vi "Read WebSocket.vi"(8 "error in (no error)":errorcluster, 11 "Connection Handler in":refnum<class "Connection Handler.lvclass">) -> (0 "error out":errorcluster, 2 "Socket":refnum<class "Socket.lvclass">, 3 "Connection Handler out":refnum<class "Connection Handler.lvclass">)   [LabVIEW 2017, in "Connection Handler.lvlib" / "Connection Handler.lvclass"]
uses:
  Connection Handler.lvclass
  <vilib>/MediaMongrels Ltd/WebSockets/Sockets/Socket/Socket.lvclass
  Connection Handler.lvclass/Connection Handler.ctl
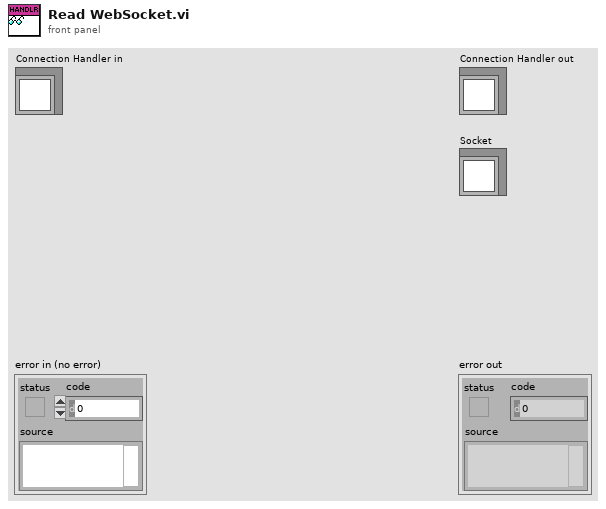
[diagram p1: front panel]
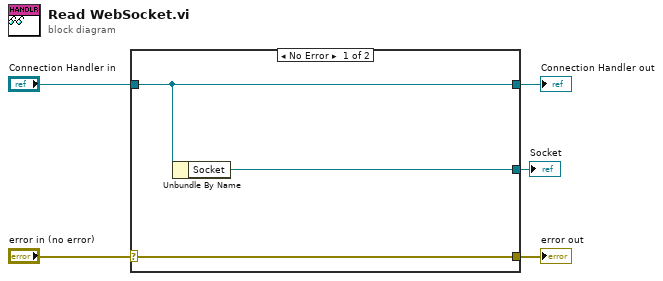
[diagram p0: block diagram]
diagram:
  n1 = case shown="No Error" "error in (no error)" {
    selector: "error in (no error)" -> [w8 w9]
    tunnel: [w8 w9] -> w4
    tunnel: [w7 w10] -> w2
    tunnel: "Connection Handler in" -> [w7 w10]
    tunnel: [w6 _] -> w1
    frame No Error {
      n2 = Unbundle By Name(w7) -> ("Socket"=w6:refnum<class "Socket.lvclass">)
    }
    frame Error {
    }
  }
  "error out" <- w4
  "Connection Handler out" <- w2
  "Socket" <- w1
